vi "Enhanced Data Plopper.vi"(0 "Roughness":T1) -> ()   [LabVIEW 2018]
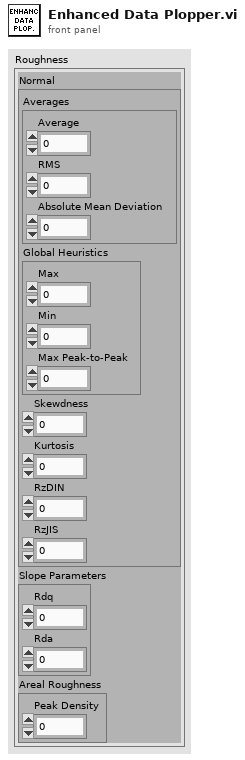
[diagram p1: front panel]
types:
  T1 = cluster{"Normal":cluster{"Averages":cluster{"Average":dbl, "RMS":dbl, "Absolute Mean Deviation":dbl}, "Global Heuristics":cluster{"Max":dbl, "Min":dbl, "Max Peak-to-Peak":dbl}, "Skewdness":dbl, "Kurtosis":dbl, "RzDIN":dbl, "RzJIS":dbl}, "Slope Parameters":cluster{"Rdq":dbl, "Rda":dbl}, "Areal Roughness":cluster{"Peak Density":dbl}}
  T2 = enum32{"Invalid", "Standard", "Closed", "Hidden", "Minimized", "Maximized"}
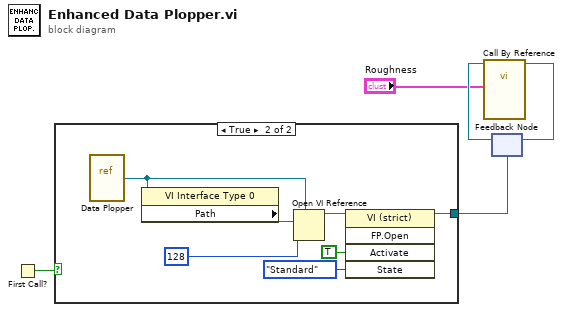
[diagram p0: block diagram]
diagram:
  n1 = First Call?() -> (First Call?: T/F=w5:bool)
  n2 = case shown="True" w5 {
    tunnel: [_ w8] -> w4
    frame False {
    }
    frame True {
      n3 = vi-ref "Data Plopper.vi"() -> (w10:refnum<vi>)
      n4 = property class="VI Interface Type 0"(reference=w10) -> ("Path"=w12:path)  [unwired: 1 in, 2 out]
      n5 = Open VI Reference(type specifier VI Refnum (for type only)=w10, vi path=w12, options=128) -> (vi reference=w9:refnum<vi>)  [unwired: 3 in, 1 out]
      n6 = invoke class="VI (strict)" method="FP.Open"(reference=w9, "Activate"=TRUE ("Activate?"), "State"=T2."Standard") -> (reference out=w8:refnum<vi>)  [unwired: 2 in, 4 out]
    }
  }
  n7 = feedback #1(w4) -> (w3:refnum<vi>)
  n8 = call-by-ref "?"(reference=w3, "Roughness"="Roughness") -> (reference out=w2:refnum<vi>)  [unwired: 12 in, 1 out]
  n9 = feedback-in #1(w2) -> ()
